vi "Write reading_timeout.vi"(8 "error in (no error)":errorcluster, 10 "reading_timeout":i32=10, 11 "TCPSettings in":refnum<class "TCPSettings.lvclass">) -> (0 "error out":errorcluster, 3 "TCPSettings out":refnum<class "TCPSettings.lvclass">)   [LabVIEW 2016, in "TCPSettings.lvclass"]
uses:
  TCPSettings.lvclass
  TCPSettings.lvclass/TCPSettings.ctl
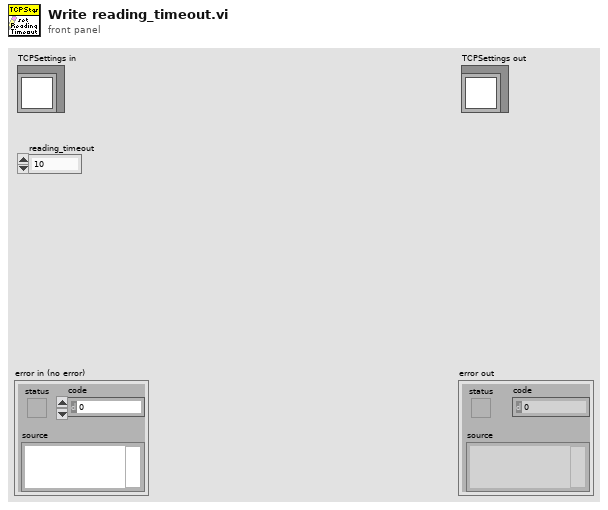
[diagram p1: front panel]
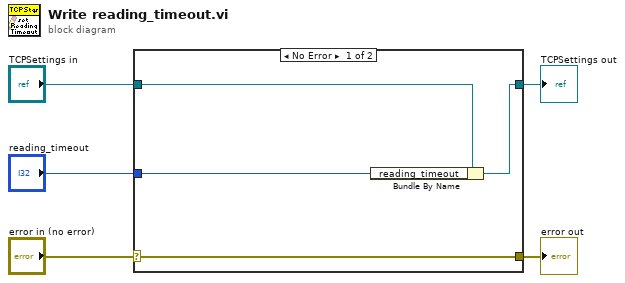
[diagram p0: block diagram]
diagram:
  n1 = case shown="No Error" "error in (no error)" {
    selector: "error in (no error)" -> [w9 w10]
    tunnel: [w9 w10] -> w4
    tunnel: [w7 w11] -> w2
    tunnel: "TCPSettings in" -> [w8 w11]
    tunnel: "reading_timeout" -> [w6 _]
    frame No Error {
      n2 = Bundle By Name(cluster=w8, "reading_timeout"=w6) -> (w7:refnum<class "TCPSettings.lvclass">)
    }
    frame Error {
    }
  }
  "error out" <- w4
  "TCPSettings out" <- w2
